vi "HVBuncher.ProcEvents.vi"(0 "i ref in":refnum<vi>, 5 "error in (no error)":errorcluster) -> (14 "i ref out":refnum<vi>, 19 "error out":errorcluster)   [LabVIEW 2014, in "HVBuncher.lvlib"]
doc: "This method is used to define the events the object will listen to. Add your own events here."
uses:
  HVBuncher.lvlib
  CS_Core/CAEObj/CAEObj.event definition.ctl
  CS_Core/BaseProcess/BaseProcess.event definition.ctl
  CS_Core/BaseProcess/BaseProcess.descriptor string definition.ctl
  CS_Core/BaseProcess/BaseProcess.lvlib
  CS_Core/CAEObj/CAEObj.lvlib
panel:
  in  "event definition type":T1
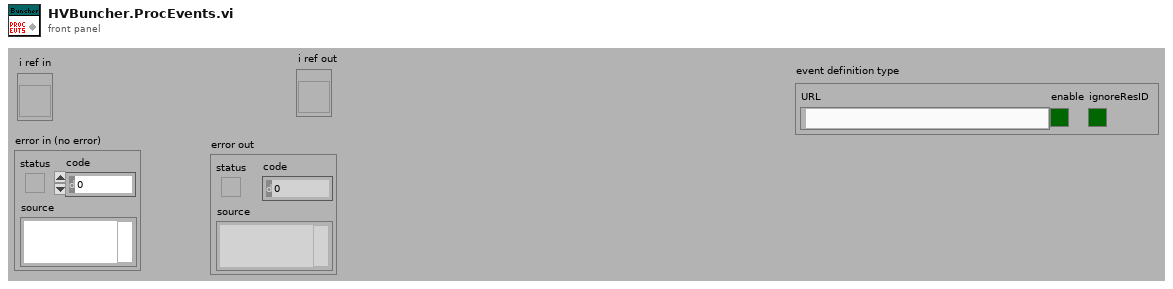
[diagram p1: front panel]
types:
  T1 = typedef "CAEObj.lvlib/CAEObj.event definition.ctl" = cluster{"URL":string, "enable":bool, "ignoreResID":bool}
  T2 = typedef "BaseProcess.lvlib/BaseProcess.event definition.ctl" = cluster{"CAEEvtDef":T1, "Data Descriptor":T3}
  T3 = typedef "BaseProcess.lvlib/BaseProcess.descriptor string definition.ctl" = string
  T4 = typedef "HVBuncher.lvlib/HVBuncher.i attribute.ctl" = cluster{"ObjectsInitialized":bool, "ChildObjects":T5}
  T5 = typedef "HVBuncher.lvlib/HVBuncher.ChildObjects.ctl" = cluster{"ObjectsLoaded":string[], "actVoltage":dbl[]}
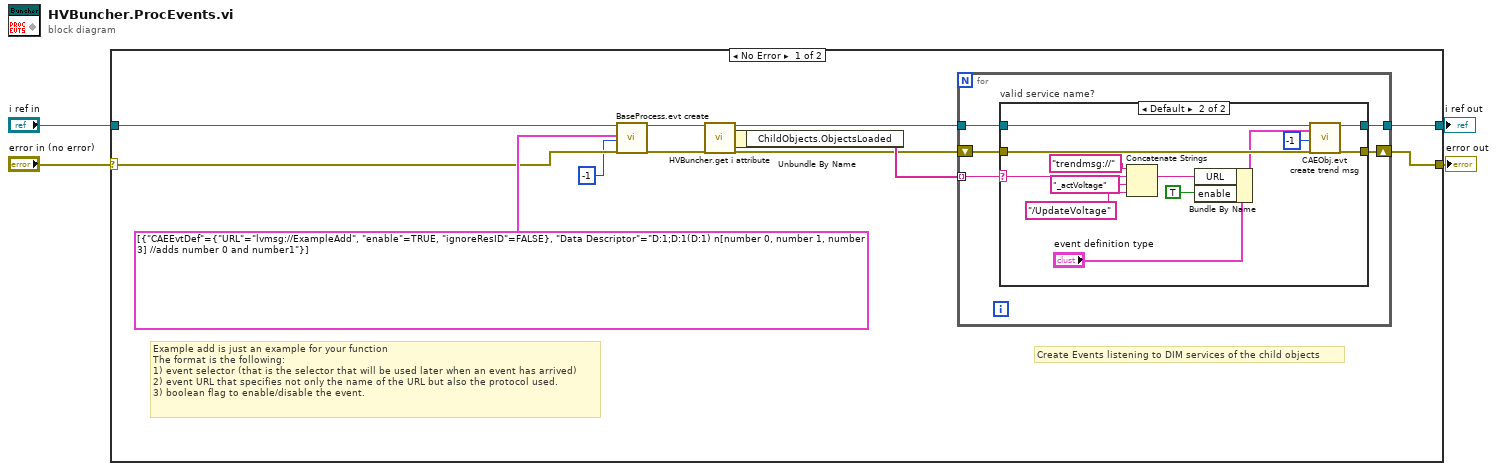
[diagram p0: block diagram]
diagram:
  n1 = case shown="No Error" "error in (no error)" {
    selector: "error in (no error)" -> [w14 w37]
    tunnel: "i ref in" -> [w16 w38]
    tunnel: [w12 w38] -> w3
    tunnel: [w11 w37] -> w2
    frame No Error {
      # "Create Events listening to DIM services of the child objects"
      # "Example add is just an example for your function\nThe format is the following:\n1) event selector (that is the selector that will be used later when an event has arrived)\n2) event URL that specifies not only the name of the URL but also the protocol used.\n3) boolean flag to enable/disable the event."
      n2 = call "BaseProcess.evt create.vi"("i ref in"=w16, "newEvents"=T2[] [{"CAEEvtDef"={"URL"="lvmsg://ExampleAdd", "enable"=TRUE, "ignoreResID"=FALSE}, "Data Descriptor"="D:1;D:1(D:1) n[number 0, number 1, number 3] //adds number 0 and number1"}] ("new events"), "ms timeout (10000)"=-1, "error in (no error)"=w14) -> ("i ref out"=w10:refnum<vi>, "error out"=w9:errorcluster)  [unwired: 12 in, 2 out]
      n3 = call "HVBuncher.get i attribute.vi"("i ref in"=w10, "error in (no error)"=w9) -> ("i ref out"=w6:refnum<vi>, "i attribute"=w8:T4, "error out"=w5:errorcluster)  [unwired: 15 in]
      n4 = Unbundle By Name(w8) -> ("ChildObjects.ObjectsLoaded"=w7:string[])
      n5 = for {
        tunnel: [w21] -> w12
        shift-right: [w20] -> w11
        shift-left: w5 -> [w18]
        tunnel: w7 -> [w19] mode=indexing
        tunnel: w6 -> [w17]
        n6 = case "valid service name?" shown="Default" w19 {
          selector: w19 -> [_ w26]
          tunnel: w17 -> [w23 w34]
          tunnel: [w23 w33] -> w21
          tunnel: w18 -> [w22 w32]
          tunnel: [w22 w31] -> w20
          frame "N/A" {
          }
          frame Default {
            n7 = Concatenate Strings("trendmsg://" ("string"), w26, "_actVoltage" ("string"), "/UpdateVoltage" ("string")) -> (w30:string)
            n8 = Bundle By Name(cluster="event definition type", "URL"=w30, "enable"=TRUE) -> (w27:T1)
            n9 = call "CAEObj.evt create trend msg.vi"("i ref in"=w34, "event definition"=w27, "ms timeout (10000)"=-1 ("ms timeout (100)"), "error in (no error)"=w32) -> ("i ref out"=w33:refnum<vi>, "error out"=w31:errorcluster)  [unwired: 12 in, 2 out]
          }
        }
      }
    }
    frame Error {
    }
  }
  "i ref out" <- w3
  "error out" <- w2
